vi "Write Audio File (Polymorphic Template).vi"   [LabVIEW 2020]
uses:
  d52d828a-60e9-43b7-91bc-9376d25dd751.vi
  807f39b4-acd1-4e10-be90-dcf34940c9e4.vi
  a5e1cc0f-5260-4a2c-ba61-69e454cee05e.vi
  8f001d3d-3eba-4621-a1dd-25cdb8a387f5.vi
  75815c75-30ff-4155-b4e1-49d7c49b6e1a.vi
  77190bfe-c304-4b37-ab79-66ef03d1b00f.vi
  b75a90c6-0968-4caf-8242-b16c6b03b6e9.vi
  63fea248-8c41-46ff-8174-b82f813d17d6.vi
  76213f91-1335-4f0b-aeec-b40707baec9b.vi
  662d7aef-f0ef-47db-b587-7f6c06629066.vi
  f99bcea3-69db-40ac-8635-f02b9e8cedc7.vi
  46e15a31-2784-4bd5-bed7-5e8cd2ec4184.vi
  96d235e9-0471-42cb-8a3a-14b043485e7e.vi
  e3e4bab6-d655-48d8-87c8-4f03097134c6.vi
  82dcce82-76fd-4bd2-9d9e-d2d8f48b9bef.vi
  33fa214b-6976-4a50-8ead-1c2edc194194.vi
  33355bcc-cb21-4921-96ac-c961374aac82.vi
  cd52ab94-533e-4246-8336-756da2cd586c.vi
  8410fdee-f49f-441d-b82b-34e35d61dd32.vi
  a6c6f6dd-d3d7-474f-8ff7-3dd6be336c07.vi
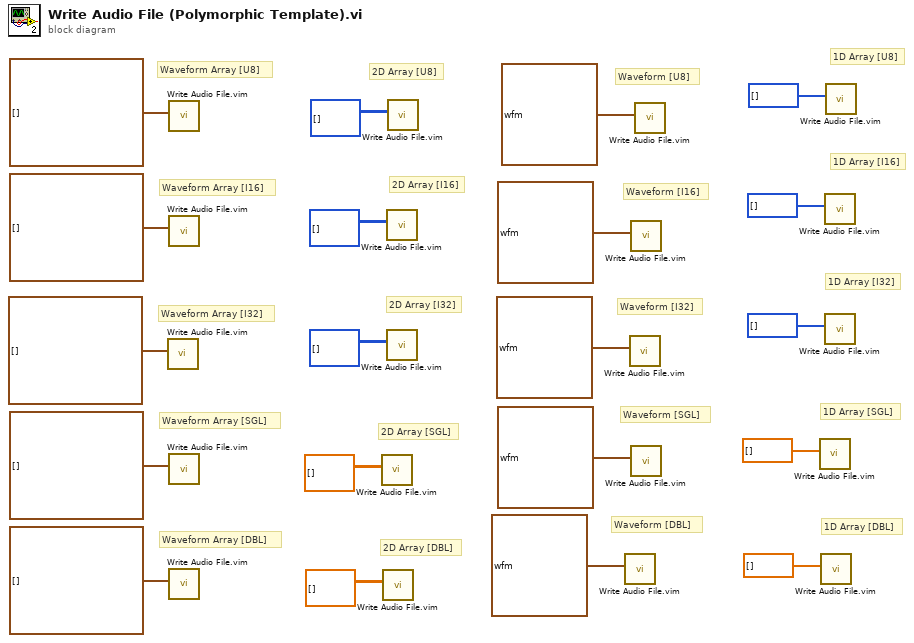
[diagram p0: block diagram]
diagram:
  # "1D Array [DBL]"
  # "1D Array [SGL]"
  # "1D Array [I32]"
  # "1D Array [I16]"
  # "1D Array [U8]"
  # "Waveform [DBL]"
  # "Waveform [SGL]"
  # "Waveform [I32]"
  # "Waveform [I16]"
  # "Waveform [U8]"
  # "2D Array [DBL]"
  # "2D Array [SGL]"
  # "2D Array [I32]"
  # "2D Array [I16]"
  # "2D Array [U8]"
  # "Waveform Array [DBL]"
  # "Waveform Array [SGL]"
  # "Waveform Array [I32]"
  # "Waveform Array [I16]"
  # "Waveform Array [U8]"
  n1 = call "Write Audio File.vim"("Audio Data"=waveform(i32)[] [] ("Data Format (I16 Waveform Array)")) -> ()  [unwired: 9 in, 2 out]
  n2 = call "Write Audio File.vim"("Audio Data"=waveform(u8)[] [] ("Data Format (I16 Waveform Array)")) -> ()  [unwired: 9 in, 2 out]
  n3 = call "Write Audio File.vim"("Audio Data"=waveform(i16)[] [] ("Data Format (I16 Waveform Array)")) -> ()  [unwired: 9 in, 2 out]
  n4 = call "Write Audio File.vim"("Audio Data"=waveform(sgl)[] [] ("Data Format (I16 Waveform Array)")) -> ()  [unwired: 9 in, 2 out]
  n5 = call "Write Audio File.vim"("Audio Data"=waveform(dbl)[] [] ("Data Format (I16 Waveform Array)")) -> ()  [unwired: 9 in, 2 out]
  n6 = call "Write Audio File.vim"("Audio Data"=sgl[][] []) -> ()  [unwired: 9 in, 2 out]
  n7 = call "Write Audio File.vim"("Audio Data"=dbl[][] []) -> ()  [unwired: 9 in, 2 out]
  n8 = call "Write Audio File.vim"("Audio Data"=i16[][] []) -> ()  [unwired: 9 in, 2 out]
  n9 = call "Write Audio File.vim"("Audio Data"=i32[][] []) -> ()  [unwired: 9 in, 2 out]
  n10 = call "Write Audio File.vim"("Audio Data"=u8[][] []) -> ()  [unwired: 9 in, 2 out]
  n11 = call "Write Audio File.vim"("Audio Data"=waveform(dbl) {"t0"=timestamp(0 s since 1904-01-01), "dt"=1.0, "Y"=[]} ("Waveform")) -> ()  [unwired: 9 in, 2 out]
  n12 = call "Write Audio File.vim"("Audio Data"=waveform(i32) {"t0"=timestamp(0 s since 1904-01-01), "dt"=1.0, "Y"=[]} ("Waveform")) -> ()  [unwired: 9 in, 2 out]
  n13 = call "Write Audio File.vim"("Audio Data"=waveform(i16) {"t0"=timestamp(0 s since 1904-01-01), "dt"=1.0, "Y"=[]} ("Waveform")) -> ()  [unwired: 9 in, 2 out]
  n14 = call "Write Audio File.vim"("Audio Data"=waveform(sgl) {"t0"=timestamp(0 s since 1904-01-01), "dt"=1.0, "Y"=[]} ("Waveform")) -> ()  [unwired: 9 in, 2 out]
  n15 = call "Write Audio File.vim"("Audio Data"=waveform(u8) {"t0"=timestamp(0 s since 1904-01-01), "dt"=1.0, "Y"=[]} ("Waveform")) -> ()  [unwired: 9 in, 2 out]
  n16 = call "Write Audio File.vim"("Audio Data"=sgl[] []) -> ()  [unwired: 9 in, 2 out]
  n17 = call "Write Audio File.vim"("Audio Data"=dbl[] []) -> ()  [unwired: 9 in, 2 out]
  n18 = call "Write Audio File.vim"("Audio Data"=i16[] []) -> ()  [unwired: 9 in, 2 out]
  n19 = call "Write Audio File.vim"("Audio Data"=i32[] []) -> ()  [unwired: 9 in, 2 out]
  n20 = call "Write Audio File.vim"("Audio Data"=u8[] []) -> ()  [unwired: 9 in, 2 out]
